vi "UHR-Fleezers Control (host) - 11.9.vi"() -> ()   [LabVIEW 2014] (continued)
                n2362 = call "IMAQ Overlay Oval"("Color"=u32 16711680, "Bounding Rectangle"=w3380, "Image"=w3383) -> ("Image Out"=w3381:T2)  [unwired: 7 in, 1 out]
              }
            }
            "Primary Video Display" <- w3352
          }
        }
        n2363 = node-c288(w3314) -> ()  [unwired: 1 out]
      }
      n2364 = node-c288(w3298) -> ()  [unwired: 1 out]
      n2365 = call "DMR_CloseDevice2.vi"("driver handle IN"=w3303) -> ()  [unwired: 1 in, 4 out]
    }
    frame #4 {
      n2366 = call "DMR_Close.vi"() -> ()  [unwired: 1 out]
    }
  }
  n2367 = local write "Offset (nm)"(0.0 ("Offset (nm)")) -> ()
  n2368 = local write "Bead Mean (nm)"(0.0 ("Bead Mean (nm)")) -> ()
  n2369 = local write "Total Volume\nFlowed P1 (uL)"(w14) -> ()
  n2370 = local write "Total Volume\nFlowed Samp (uL)"(w14) -> ()
  n2371 = local write "Total Volume\nFlowed P3 (uL)"(w14) -> ()
  n2372 = node-c288(i64 1 ("Period"), 1 ("Processor")) -> (w193:T21)  [unwired: 2 out]
  n2373 = timed-loop "Acquire Data" {
    tunnel: w20 -> [w3749]
    tunnel: w69 -> [w3748]
    tunnel: [w3778] -> w286
    tunnel: [w3773] -> w284
    timing: w193 -> [_]
    timing-out: [_] -> w192
    tunnel: w88 -> [w3588]
    stop <- "Stop All" stop-if-true
    w3506 = "Initialize"
    w3575 = "NI_ChannelName" ("name")
    # "I think that the conversion\nfrom 'wiggle amp' to nm\nis 0.277 nm/input. So, 1000\nfor an input is 277 nm."
    n2374 = node-c288() -> ()  [unwired: 2 out]
    n2375 = First Call?() -> (First Call?: T/F=w3541:bool)
    n2376 = Or(x="Reset", y=w3541) -> (x .or. y?=w3542:bool)
    n2377 = local read "Flushing P1"() -> (w3461:bool)
    n2378 = case "Reset data stream" shown="True" w3542 {
      tunnel: w3749 -> [w4816 w4824]
      tunnel: w3748 -> [w4815 w4823]
      tunnel: [w4816 w4818] -> w3454
      tunnel: [w4815 w4817] -> w3744
      frame False {
      }
      frame True {
        w4821 = TRUE ("AI to FIFO")
        n2379 = local write "Overflow (data lost)"(FALSE ("Overflow (data lost)")) -> ()
        n2380 = call "reset FPGA DMA.vi"("error in"=w4823, "FPGA VI Reference In"=w4824) -> ("error out"=w4819:errorcluster, "FPGA VI Reference Out"=w4820:T19)
        n2381 = xnode "Read/Write Control"("FPGA VI Reference In"=w4820, "error in"=w4819, "AI to FIFO"=w4821, "APD to FIFO"=w4821) -> ("FPGA VI Reference Out"=w4818:T19, "error out"=w4817:errorcluster)
      }
    }
    n2382 = case shown="True" w3461 {
      frame False {
      }
      frame True {
        n2383 = local read "Flush rate (uL/m) P1"() -> (w3851:dbl)
        n2384 = local read "HP1 Flush Time (s)"() -> (w3857:dbl)
        n2385 = local read "DMA Update Period (s)"() -> (w3844:dbl)
        n2386 = Divide(x=w3851, y=60.0) -> (x/y=w3843:dbl)
        n2387 = feedback #4(0.0) -> (w3846:dbl)
        n2388 = Divide(x=w3857, y=w3844) -> (x/y=w3849:dbl)
        n2389 = feedback #5(0) -> (w3855:i32)
        n2390 = Increment(x=w3855) -> (x+1=w3848:i32)
        n2391 = Multiply(x=w3844, y=w3843) -> (x*y=w3842:dbl)
        n2392 = Greater?(x=w3848, y=w3849) -> (0:w3854:bool)
        n2393 = Compound Arithmetic op=MULTIPLY(w3844, w3848, w3843) -> (→"P1 Flush Volume (uL)":dbl)
        n2394 = Divide(x=w3848, y=w3849) -> (x/y=→"P1 Flushing Bar":dbl)
        n2395 = Add(x=w3842, y=w3846) -> (x+y=w3845:dbl)
        "Total Volume\nFlowed P1 (uL)" <- w3845
        n2396 = feedback-in #4(w3845) -> ()
        n2397 = case shown="True" w3854 {
          tunnel: w3848 -> [w3858 _]
          tunnel: [w3858 0] -> w3853
          frame False {
          }
          frame True {
            w3859 = FALSE ("Flushing P1")
            n2398 = local write "Inject Pump 1"(w3859) -> ()
            n2399 = local write "Flushing P1"(w3859) -> ()
            n2400 = property on="Clear Volume P1" class="Bool (strict)"("Val(Sgnl)"=TRUE ("Value (Signaling)")) -> ()  [unwired: 2 in, 2 out]
          }
        }
        n2401 = feedback-in #5(w3853) -> ()
      }
    }
    n2402 = Or(x="Start AOD Scan", y="Trap Raster Scan") -> (x .or. y?=w3696:bool)
    n2403 = case "Start AOM raster scan" shown="True" w3696 {
      tunnel: w3454 -> [w4666 w4676]
      tunnel: w3744 -> [w4665 w4675]
      tunnel: [w4666 w4669] -> w3446
      tunnel: [w4665 w4668] -> w3743
      frame False {
      }
      frame True {
        n2404 = case shown="True" "Restart DMA? (AOD)" {
          tunnel: [w4714 w4716] -> w4670
          tunnel: [w4713 w4715] -> w4671
          tunnel: w4676 -> [w4714 w4718]
          tunnel: w4675 -> [w4713 w4717]
          frame False {
          }
          frame True {
            n2405 = local write "Overflow (data lost)"(FALSE ("Overflow (data lost)")) -> ()
            n2406 = call "reset FPGA DMA.vi"("error in"=w4717, "FPGA VI Reference In"=w4718) -> ("error out"=w4715:errorcluster, "FPGA VI Reference Out"=w4716:T19)
          }
        }
        n2407 = local write "Trap Raster Scan"(FALSE ("Trap Raster Scan")) -> ()
        n2408 = case shown="False" "Move MCL Also?" {
          tunnel: w4671 -> [w4680 w4708]
          tunnel: w4670 -> [w4681 w4709]
          tunnel: [w4679 w4712] -> w4669
          tunnel: [w4678 w4711] -> w4668
          frame False {
            w4677 = TRUE ("AI to FIFO")
            n2409 = xnode "Read/Write Control"("FPGA VI Reference In"=w4681, "error in"=w4680, "AI to FIFO"=w4677, "APD to FIFO"=w4677, "Start scan"=w4677) -> ("FPGA VI Reference Out"=w4679:T19, "error out"=w4678:errorcluster)
          }
          frame True {
            w4705 = FALSE ("1D or 2D Scan?")
            w4710 = TRUE ("AI to FIFO")
            # "Count for MCL loop"
            # "N total cycles"
            # "N steps"
            # "V_int"
            n2410 = local read "Scan Range (nm)"() -> (w4687:dbl)
            n2411 = local read "Number of F/B Scans (AOD)"() -> (w4704:u16)
            n2412 = Sign(1:w4687) -> (0:w4686:dbl)
            n2413 = Compound Arithmetic op=MULTIPLY(w4687, "MCL Step Position Ratio", "MCL/AOM Scale Tweak") -> (w4691:dbl)
            n2414 = Negate(x=w4686) -> (-x=w4683:dbl)
            n2415 = Multiply(x=w4683, y="MCL Step Increment (V_int)") -> (x*y=w4685:dbl)
            n2416 = Divide(x=w4691, y="MCL X Cal (nm/V)") -> (x/y=w4697:dbl)
            n2417 = Multiply(x=32767.0 ("y"), y=w4697) -> (x*y=w4703:dbl)
            n2418 = local read "Total Counts (ticks)"() -> (w4688:u32)
            n2419 = local read "Cycles/step (AOD)"() -> (w4699:u64)
            n2420 = local read "Scan steps (AOD)"() -> (w4700:u64)
            n2421 = Divide(x=w4703, y=10.0) -> (x/y=w4696:dbl)
            n2422 = Divide(x=w4696, y="MCL Step Increment (V_int)") -> (x/y=w4694:dbl)
            n2423 = Absolute Value(x=w4694) -> (abs(x)=w4682:dbl)
            n2424 = Compound Arithmetic op=MULTIPLY(w4700, w4699, w4688) -> (w4695:u64)
            n2425 = local write "wait to reset values"(w4710) -> ()
            n2426 = local write "MCL Scanning"(w4710) -> ()
            n2427 = Divide(x=w4695, y=w4682) -> (x/y=w4692:dbl)
            "MCL Count" <- w4692
            n2428 = xnode "Read/Write Control"("FPGA VI Reference In"=w4709, "error in"=w4708, "Scan steps (MCL)"=w4682, "Number of scans (MCL)"=w4704, "Cycles per step (MCL)"=u64 1, "Scan freq.  increment (MCL)"=w4685, "1D or 2D Scan?"=w4705, "MCL Scan Axis"=w4705, "Cont. Scan (MCL)"=w4705, "MCL count"=w4692) -> ("FPGA VI Reference Out"=w4707:T19, "error out"=w4706:errorcluster)
            n2429 = xnode "Read/Write Control"("FPGA VI Reference In"=w4707, "error in"=w4706, "AI to FIFO"=w4710, "APD to FIFO"=w4710, "Start scan"=w4710, "Start scan (MCL)"=w4710) -> ("FPGA VI Reference Out"=w4712:T19, "error out"=w4711:errorcluster)
          }
        }
        "Raster Scanning..." <- TRUE ("Scanning...")
      }
    }
    n2430 = local read "Flushing P3"() -> (w3462:bool)
    n2431 = case "Keep track of when Harvard Pump 3 is done flushing" shown="True" w3462 {
      frame False {
      }
      frame True {
        n2432 = local read "Flush rate (uL/m) P3"() -> (w3870:dbl)
        n2433 = local read "DMA Update Period (s)"() -> (w3864:dbl)
        n2434 = local read "HP3 Flush Time (s)"() -> (w3878:dbl)
        n2435 = Divide(x=w3870, y=60.0) -> (x/y=w3865:dbl)
        n2436 = feedback #6(0) -> (w3876:i32)
        n2437 = Increment(x=w3876) -> (x+1=w3871:i32)
        n2438 = Divide(x=w3878, y=w3864) -> (x/y=w3872:dbl)
        n2439 = Multiply(x=w3864, y=w3865) -> (x*y=w3863:dbl)
        n2440 = Greater?(x=w3871, y=w3872) -> (0:w3875:bool)
        n2441 = feedback #7(0.0) -> (w3866:dbl)
        n2442 = Compound Arithmetic op=MULTIPLY(w3864, w3871, w3865) -> (→"P3 Flush Volume (uL)":dbl)
        n2443 = case shown="True" w3875 {
          tunnel: w3871 -> [w3879 _]
          tunnel: [w3879 0] -> w3874
          frame False {
          }
          frame True {
            w3880 = FALSE ("Flushing P3")
            n2444 = local write "Inject Pump 3"(w3880) -> ()
            n2445 = local write "Flushing P3"(w3880) -> ()
            n2446 = property on="Clear Volume P3" class="Bool (strict)"("Val(Sgnl)"=TRUE ("Value (Signaling)")) -> ()  [unwired: 2 in, 2 out]
          }
        }
        n2447 = feedback-in #6(w3874) -> ()
        n2448 = Divide(x=w3871, y=w3872) -> (x/y=→"P3 Flushing Bar":dbl)
        n2449 = Add(x=w3863, y=w3866) -> (x+y=w3867:dbl)
        "Total Volume\nFlowed P3 (uL)" <- w3867
        n2450 = feedback-in #7(w3867) -> ()
      }
    }
    n2451 = And(x="Save scans", y=w3696) -> (x .and. y?=w3742:bool)
    n2452 = local read "Flushing samp"() -> (w3455:bool)
    n2453 = case shown="True" w3455 {
      frame False {
      }
      frame True {
        n2454 = local read "DMA Update Period (s)"() -> (w3823:dbl)
        n2455 = local read "Flush rate (mL/m)"() -> (w3835:dbl)
        n2456 = local read "Samp Flush Time (s)"() -> (w3836:dbl)
        n2457 = Divide(x=w3835, y=60.0) -> (x/y=w3822:dbl)
        n2458 = feedback #8(0) -> (w3828:i32)
        n2459 = Increment(x=w3828) -> (x+1=w3827:i32)
        n2460 = Divide(x=w3836, y=w3823) -> (x/y=w3832:dbl)
        n2461 = Multiply(x=w3823, y=w3822) -> (x*y=w3821:dbl)
        n2462 = Greater?(x=w3827, y=w3832) -> (0:w3831:bool)
        n2463 = feedback #9(0.0) -> (w3824:dbl)
        n2464 = Compound Arithmetic op=MULTIPLY(w3823, w3827, w3822) -> (→"Samp Volume (uL)":dbl)
        n2465 = Divide(x=w3827, y=w3832) -> (x/y=→"Samp flush bar":dbl)
        n2466 = case shown="True" w3831 {
          tunnel: [w3837 0] -> w3830
          tunnel: w3827 -> [w3837 _]
          frame False {
          }
          frame True {
            w3840 = FALSE ("Flushing samp")
            n2467 = local write "Sample Channel\nFlow"(w3840) -> ()
            n2468 = local write "Flushing samp"(w3840) -> ()
            n2469 = property on="Clear Volume" class="Bool (strict)"("Val(Sgnl)"=TRUE) -> ()  [unwired: 2 in, 2 out]
          }
        }
        n2470 = feedback-in #8(w3830) -> ()
        n2471 = Add(x=w3821, y=w3824) -> (x+y=w3825:dbl)
        "Total Volume\nFlowed Samp (uL)" <- w3825
        n2472 = feedback-in #9(w3825) -> ()
      }
    }
    n2473 = Compound Arithmetic op=OR("Start MCL Scan", "Confocal\nImage", "Confocal\nLinescan") -> (w3694:bool)
    n2474 = And(x="Save Data (MCL)", y=w3694) -> (x .and. y?=w3741:bool)
    n2475 = case "Start MCL raster scan" shown="True" w3694 {
      tunnel: w3446 -> [w4283 w4299]
      tunnel: w3743 -> [w4282 w4298]
      tunnel: [w4283 w4294] -> w3453
      tunnel: [w4282 w4293] -> w3451
      tunnel: [FALSE w4292] -> w3727
      tunnel: "Start MCL Scan" -> [_ w4287]
      tunnel: "Confocal\nImage" -> [_ w4286]
      tunnel: "Confocal\nLinescan" -> [_ _]
      frame False {
      }
      frame True {
        w4292 = TRUE
        n2476 = case shown="True" "Restart DMA? (MCL)" {
          tunnel: [w4344 w4346] -> w4297
          tunnel: [w4343 w4345] -> w4296
          tunnel: w4299 -> [w4344 w4349]
          tunnel: w4298 -> [w4343 w4348]
          frame False {
          }
          frame True {
            n2477 = call "reset FPGA DMA.vi"("error in"=w4348, "FPGA VI Reference In"=w4349) -> ("error out"=w4345:errorcluster, "FPGA VI Reference Out"=w4346:T19)
            n2478 = local write "Overflow (data lost)"(FALSE ("Overflow (data lost)")) -> ()
          }
        }
        n2479 = case shown="False" w4287 {
          selector: w4287 -> [_ w4303]
          tunnel: w4286 -> [w4302 _]
          tunnel: [w4302 w4303] -> w4285
          frame False {
            n2480 = property on="2D or 1D Scan" class="Bool (strict)"("Val(Sgnl)"=w4302) -> ()  [unwired: 2 in, 2 out]
            n2481 = property on="Confocal\nImage" class="Bool (strict)"("Value"=FALSE ("Start Confocal Map")) -> ()  [unwired: 2 in, 2 out]
          }
          frame True {
          }
        }
        n2482 = local write "MCL Scanning"(w4292) -> ()
        n2483 = local read "AO1"() -> (w4289:dbl)
        n2484 = local read "AO2"() -> (w4288:dbl)
        n2485 = case shown="True" "Center Scan" {
          tunnel: w4297 -> [w4310 w4342]
          tunnel: w4296 -> [w4309 w4341]
          tunnel: [w4308 w4340] -> w4294
          tunnel: [w4307 w4339] -> w4293
          tunnel: [w4305 w4326] -> w4291
          tunnel: [w4304 w4325] -> w4290
          tunnel: w4289 -> [w4305 w4331]
          tunnel: w4288 -> [w4304 w4334]
          tunnel: w4285 -> [_ _]
          frame False {
            w4306 = TRUE ("AI to FIFO")
            n2486 = xnode "Read/Write Control"("FPGA VI Reference In"=w4310, "error in"=w4309, "AI to FIFO"=w4306, "APD to FIFO"=w4306, "Start scan (MCL)"=w4306) -> ("FPGA VI Reference Out"=w4308:T19, "error out"=w4307:errorcluster)
          }
          frame True {
            w4338 = TRUE ("AI to FIFO")
            n2487 = local read "Scan steps (MCL)"() -> (w4317:u64)
            n2488 = local read "Scan lines (y)"() -> (w4313:u64)
            n2489 = local read "Fast Scan Dir"() -> (w4324:bool)
            n2490 = local read "Actual MCL Inc (V)"() -> (w4314:dbl)
            n2491 = Decrement(x=w4313) -> (x-1=w4312:u64)
            n2492 = Decrement(x=w4317) -> (x-1=w4316:u64)
            n2493 = Multiply(x=w4314, y=w4312) -> (x*y=w4311:dbl)
            n2494 = Divide(x=w4311, y=2.0) -> (x/y=w4321:dbl)
            n2495 = Multiply(x=w4314, y=w4316) -> (x*y=w4315:dbl)
            n2496 = Divide(x=w4315, y=2.0) -> (x/y=w4320:dbl)
            n2497 = Select(t=w4320, s=w4324, f=w4321) -> (s? t:f=w4319:dbl)
            n2498 = Select(t=w4321, s=w4324, f=w4320) -> (s? t:f=w4323:dbl)
            n2499 = Subtract(x=w4331, y=w4323) -> (x-y=w4322:dbl)
            n2500 = Subtract(x=w4334, y=w4319) -> (x-y=w4318:dbl)
            n2501 = local read "2D or 1D Scan"() -> (w4336:bool)
            n2502 = Not(x=w4324) -> (.not. x?=w4330:bool)
            n2503 = Not(x=w4336) -> (.not. x?=w4332:bool)
            n2504 = And(x=w4324, y=w4332) -> (x .and. y?=w4333:bool)
            n2505 = And(x=w4332, y=w4330) -> (x .and. y?=w4335:bool)
            n2506 = Select(t=w4334, s=w4335, f=w4318) -> (s? t:f=w4325:dbl)
            n2507 = Select(t=w4331, s=w4333, f=w4322) -> (s? t:f=w4326:dbl)
            n2508 = call "Volt to I16.vi"("Voltage In"=w4326) -> ("I16 Voltage Out"=w4329:i16)
            n2509 = call "Volt to I16.vi"("Voltage In"=w4325) -> ("I16 Voltage Out"=w4328:i16)
            n2510 = xnode "Read/Write Control"("FPGA VI Reference In"=w4342, "error in"=w4341, "AI to FIFO"=w4338, "APD to FIFO"=w4338, "Start scan (MCL)"=w4338, "AO1"=w4329, "AO2"=w4328) -> ("FPGA VI Reference Out"=w4340:T19, "error out"=w4339:errorcluster)
          }
        }
        "Initial Y" <- w4291
        "Initial X" <- w4290
        n2511 = local write "Tab Control 6"(T3."Imaging" ("Tab Control 6")) -> ()
        "wait to reset values" <- w4292
      }
    }
    n2512 = xnode "Read/Write Control"("FPGA VI Reference In"=w3446) -> ("Green Enabled"=w3445)  [unwired: 1 in, 2 out]
    n2513 = local write "Grn enabl"(w3445) -> ()
    n2514 = case shown="True" "Wiggle" {
      selector: "Wiggle" -> [w3794 _]
      tunnel: w3453 -> [w3796 w3809]
      tunnel: [w3793 w3812] -> w3452
      tunnel: w3451 -> [w3795 w3807]
      tunnel: [w3792 w3811] -> w3450
      frame False {
        n2515 = xnode "Read/Write Control"("FPGA VI Reference In"=w3796, "error in"=w3795, "Wiggle trap 1"=w3794) -> ("FPGA VI Reference Out"=w3793:T19, "error out"=w3792:errorcluster)
      }
      frame True {
        w3801 = FALSE ("Abort wiggle")
        w3805 = TRUE
        n2516 = local read "Restart DMA? (AOD)"() -> (w3810:bool)
        n2517 = case shown="True" w3810 {
          tunnel: w3809 -> [w3814 w3819]
          tunnel: [w3814 w3818] -> w3808
          tunnel: w3807 -> [w3813 w3817]
          tunnel: [w3813 w3816] -> w3806
          frame False {
          }
          frame True {
            n2518 = local write "Overflow (data lost)"(FALSE) -> ()
            n2519 = call "reset FPGA DMA.vi"("error in"=w3817, "FPGA VI Reference In"=w3819) -> ("error out"=w3816:errorcluster, "FPGA VI Reference Out"=w3818:T19)
          }
        }
        n2520 = local write "Wiggle"(FALSE) -> ()
        n2521 = xnode "Read/Write Control"("FPGA VI Reference In"=w3808, "error in"=w3806, "AI to FIFO"=w3805, "APD to FIFO"=w3805, "Wiggle trap 1"="Wiggle T1", "Wiggle freq 1 (Hz)"="Wiggle freq 1 (Hz)", "Wiggle amp 1"="Wiggle amp 1 (units?)", "Abort wiggle 1"=w3801, "Wiggle trap 2"="Wiggle T2", "Abort wiggle 2"=w3801, "Wiggle freq 2 (Hz)"="Wig Freq 2 (Hz)", "Wiggle amp 2"="Wig amp 2") -> ("FPGA VI Reference Out"=w3812:T19, "error out"=w3811:errorcluster)
      }
    }
    n2522 = local read "Trap Pos Elements/DMA read"() -> (w3584:u32)
    n2523 = local read "Trap AI Elements/DMA read"() -> (w3657:u32)
    n2524 = local read "APD Elements/DMA read"() -> (w3623:u32)
    n2525 = xnode "Get APD Data"("FPGA VI Reference In"=w3452, "error in"=w3450, "Number of Elements"=w3623, "Timeout (ms)"=-1) -> ("Data"=w3622:u32[], "Elements Remaining"=→"APD FIFO Elements Remaining":u32)  [unwired: 2 out]
    n2526 = xnode "Invoke Method"("FPGA VI Reference In"=w3452, "error in"=w3450, "Number of Elements"=w3584, "Timeout (ms)"=-1) -> ("Data"=w3548:u16[], "Elements Remaining"=→"Trap Pos FIFO El Remaining":u32)  [unwired: 2 out]
    n2527 = xnode "Get Trap Data"("FPGA VI Reference In"=w3452, "error in"=w3450, "Number of Elements"=w3657, "Timeout (ms)"=-1 ("Timeout")) -> ("FPGA VI Reference Out"=w3483:T19, "error out"=w3482:errorcluster, "Data"=w3549:i16[], "Elements Remaining"=w3786:u32)
    "FIFO El. Rem." <- w3786
    n2528 = local read "Trap AI FIFO Depth"() -> (w3788:u32)
    n2529 = Subtract(x=w3788, y=w3657) -> (x-y=w3787:u32)
    n2530 = Decimate 1D Array(w3548) -> (w3545:u16[], w3547:u16[], w3546:u16[])
    n2531 = Divide(x=w3786, y=w3787) -> (x/y=w3785:dbl)
    "Buffer Status" <- w3785
    n2532 = To Unsigned Long Integer(number=w3545) -> (unsigned 32bit integer=w3544:u32[])
    n2533 = Join Numbers(hi=w3547, lo=w3546) -> ((hi.lo)=w3543:u32[])
    n2534 = Equal?(x=w3785, y=1.0) -> (x = y?=w3783:bool)
    n2535 = Join Numbers(hi=w3544, lo=w3543) -> ((hi.lo)=w3537:u64[])
    n2536 = call "IR AOM word to freq - vec.vi"("Frequency Word In (double vec)"=w3537) -> ("Frequency Out"=w3583:dbl[])
    n2537 = case "Alert buffer overflow" shown="True" w3783 {
      frame False {
      }
      frame True {
        n2538 = call <vilib>:"Beep.vi"() -> ()  [unwired: 3 in, 9 out]
        "Overflow (data lost)" <- TRUE ("Overflow (data lost)")
      }
    }
    n2539 = Decimate 1D Array(w3583) -> (w3582:dbl[], w3581:dbl[])
    n2540 = Build Array(w3582, w3581) -> (w3580:dbl[][])
    n2541 = local read "Trap Sets"() -> (w3656:u32)
    n2542 = case "Deinterlace trap data, average down PSD" shown="2" w3656 {
      tunnel: w3549 -> [w4379 w4444]
      tunnel: [w4376 w4441] -> w3649
      tunnel: [w4379 w4443] -> w3540
      tunnel: "Detector Type" -> [w4378 w4439]
      tunnel: [w4377 w4442] -> w3648
      tunnel: [w4375 w4440] -> w3760
      frame 1, Default {
        n2543 = Divide(x=w4379, y=3276.7) -> (x/y=w4380:dbl[])
        n2544 = Decimate 1D Array(w4380) -> (w4389:dbl[], w4388:dbl[], w4387:dbl[], w4386:dbl[], w4385:dbl[], w4384:dbl[], w4383:dbl[], w4382:dbl[])
        n2545 = case shown="\"IR-QPD + PSD + FB-QPD position\"" w4378 {
          tunnel: w4389 -> [w4413 w4438]
          tunnel: w4388 -> [w4412 w4437]
          tunnel: w4387 -> [w4397 w4415]
          tunnel: w4386 -> [w4398 w4425]
          tunnel: w4385 -> [w4411 w4436]
          tunnel: w4384 -> [w4410 w4435]
          tunnel: w4383 -> [w4394 w4416]
          tunnel: w4382 -> [w4393 w4414]
          tunnel: [w4392 w4422] -> w4377
          tunnel: [w4391 w4421] -> w4376
          tunnel: [w4390 w4420] -> w4375
          frame "IR-QPD + PSD + FB-QPD", Default {
            w4390 = 0  # Channel pattern
            n2546 = Divide(x=w4413, y=w4398) -> (x/y=w4400:dbl[])
            n2547 = Divide(x=w4412, y=w4398) -> (x/y=w4399:dbl[])
            n2548 = Divide(x=w4411, y=w4394) -> (x/y=w4396:dbl[])
            n2549 = Divide(x=w4410, y=w4393) -> (x/y=w4395:dbl[])
            n2550 = Build Array(w4400, w4399, w4398, w4397, w4396, w4395, w4394, w4393) -> (w4391:dbl[][])
            n2551 = Bundle("T1 Y", "T1 X", "T1 Sum", "FB Sum", "PSD Y", "PSD X", "PSD Y Sum", "PSD X Sum") -> (w4409:T41)  [unwired: 1 out]
            n2552 = Cluster To Array(cluster=w4409) -> (array=w4392:string[])
          }
          frame "IR-QPD + PSD + FB-QPD position" {
            w4420 = 3  # Channel pattern
            n2553 = Negate(x=w4416) -> (-x=w4417:dbl[])
            n2554 = Divide(x=w4438, y=w4425) -> (x/y=w4427:dbl[])
            n2555 = Divide(x=w4437, y=w4425) -> (x/y=w4426:dbl[])
            n2556 = Divide(x=w4436, y=w4416) -> (x/y=w4424:dbl[])
            n2557 = Divide(x=w4435, y=w4417) -> (x/y=w4423:dbl[])
            n2558 = Build Array(w4427, w4426, w4425, w4414, w4415, w4424, w4423, w4416) -> (w4421:dbl[][])
            n2559 = Bundle("T1 Y", "T1 X", "T1 Sum", "FB X", "FB Sum", "PSD Y", "PSD X", "PSD Y Sum") -> (w4434:T41)  [unwired: 1 out]
            n2560 = Cluster To Array(cluster=w4434) -> (array=w4422:string[])
          }
        }
      }
      frame 2 {
        n2561 = case shown="\"IR-QPD + PSD + FB-QPD\", Default" w4439 {
          tunnel: w4444 -> [w4506 w4573 w4644]
          tunnel: [w4445 w4564 w4575] -> w4443
          tunnel: [w4472 w4555 w4622] -> w4442
          tunnel: [w4471 w4518 w4589] -> w4441
          tunnel: [w4465 w4553 w4620] -> w4440
          frame "IR-QPD + PSD + FB-QPD", Default {
            w4465 = 1  # Channel pattern
            # "time average x2 the 4th signal and the 4 psd signals (detection laser)"
            # "deinterlace 3 signals from qpd"
            n2562 = Decimate 1D Array(w4506) -> (w4505:i16[], w4504:i16[], w4470:i16[], w4503:i16[], w4493:i16[], w4491:i16[], w4490:i16[], w4488:i16[])
            n2563 = Decimate 1D Array(w4470) -> (w4469:i16[], w4468:i16[])
            n2564 = Decimate 1D Array(w4505) -> (w4502:i16[], w4474:i16[])
            n2565 = Decimate 1D Array(w4504) -> (w4501:i16[], w4499:i16[])
            n2566 = Decimate 1D Array(w4503) -> (w4500:i16[], w4498:i16[])
            n2567 = call "downsample 1D array - double.vi"("Ave N"=2.0, "Array In"=w4493) -> ("Array Out"=w4492:dbl[])  [unwired: 1 out]
            n2568 = call "downsample 1D array - double.vi"("Ave N"=2.0, "Array In"=w4491) -> ("Array Out"=w4473:dbl[])  [unwired: 1 out]
            n2569 = call "downsample 1D array - double.vi"("Ave N"=2.0, "Array In"=w4490) -> ("Array Out"=w4489:dbl[])  [unwired: 1 out]
            n2570 = call "downsample 1D array - double.vi"("Ave N"=2.0, "Array In"=w4488) -> ("Array Out"=w4487:dbl[])  [unwired: 1 out]
            n2571 = Interleave 1D Arrays(w4502, w4501, w4500, w4474, w4499, w4498, w4469, w4468, w4492, w4473, w4489, w4487) -> (w4486:dbl[])
            n2572 = Divide(x=w4486, y=3276.7) -> (x/y=w4485:dbl[])
            n2573 = Decimate 1D Array(w4485) -> (w4484:dbl[], w4483:dbl[], w4482:dbl[], w4481:dbl[], w4480:dbl[], w4479:dbl[], w4467:dbl[], w4466:dbl[], w4478:dbl[], w4477:dbl[], w4476:dbl[], w4475:dbl[])
            n2574 = Divide(x=w4484, y=w4482) -> (x/y=w4452:dbl[])
            n2575 = Divide(x=w4483, y=w4482) -> (x/y=w4451:dbl[])
            n2576 = Divide(x=w4481, y=w4479) -> (x/y=w4450:dbl[])
            n2577 = Divide(x=w4480, y=w4479) -> (x/y=w4449:dbl[])
            n2578 = Divide(x=w4478, y=w4476) -> (x/y=w4448:dbl[])
            n2579 = Divide(x=w4477, y=w4475) -> (x/y=w4447:dbl[])
            n2580 = Build Array(w4452, w4451, w4482, w4450, w4449, w4479, w4467, w4466, w4448, w4447, w4476, w4475) -> (w4471:dbl[][])
            n2581 = Bundle("T1 Y", "T1 X", "T1 Sum", "T2 Y", "T2 X", "T2 Sum", "T1 FB Sum", "T2 FB Sum", "PSD Y", "PSD X", "PSD Y Sum", "PSD X Sum") -> (w4453:T42)  [unwired: 1 out]
            n2582 = To Word Integer(number=w4486) -> (16bit integer=w4445:i16[])
            n2583 = Cluster To Array(cluster=w4453) -> (array=w4472:string[])
          }
          frame "IR-QPD + PSD + FB-QPD X position" {
            w4553 = 2  # Channel pattern
            # "time average x2 the 3 psd signals (detection laser)"
            # "deinterlace 3 signals from qpds"
            n2584 = Decimate 1D Array(w4573) -> (w4572:i16[], w4571:i16[], w4554:i16[], w4570:i16[], w4516:i16[], w4513:i16[], w4510:i16[], w4541:i16[])
            n2585 = Decimate 1D Array(w4554) -> (w4539:i16[], w4537:i16[])
            n2586 = Decimate 1D Array(w4572) -> (w4569:i16[], w4556:i16[])
            n2587 = Decimate 1D Array(w4571) -> (w4568:i16[], w4566:i16[])
            n2588 = Decimate 1D Array(w4570) -> (w4567:i16[], w4565:i16[])
            n2589 = Decimate 1D Array(w4541) -> (w4540:i16[], w4538:i16[])
            n2590 = call "downsample 1D array - I16.vi"("Ave N"=2.0, "Array In"=w4516) -> ("Array Out"=w4514:i16[])  [unwired: 1 in]
            n2591 = call "downsample 1D array - I16.vi"("Ave N"=2.0, "Array In"=w4510) -> ("Array Out"=w4508:i16[])  [unwired: 1 in]
            n2592 = call "downsample 1D array - I16.vi"("Ave N"=2.0, "Array In"=w4513) -> ("Array Out"=w4511:i16[])  [unwired: 1 in]
            n2593 = Interleave 1D Arrays(w4569, w4568, w4567, w4556, w4566, w4565, w4540, w4539, w4538, w4537, w4514, w4511, w4508) -> (w4564:i16[])
            n2594 = Divide(x=w4564, y=3276.7) -> (x/y=w4563:dbl[])
            n2595 = Decimate 1D Array(w4563) -> (w4562:dbl[], w4561:dbl[], w4560:dbl[], w4559:dbl[], w4558:dbl[], w4557:dbl[], w4529:dbl[], w4527:dbl[], w4526:dbl[], w4524:dbl[], w4523:dbl[], w4522:dbl[], w4519:dbl[])
            n2596 = Negate(x=w4519) -> (-x=w4517:dbl[])
            n2597 = Divide(x=w4523, y=w4519) -> (x/y=w4521:dbl[])
            n2598 = Divide(x=w4522, y=w4517) -> (x/y=w4520:dbl[])
            n2599 = Divide(x=w4562, y=w4560) -> (x/y=w4545:dbl[])
            n2600 = Divide(x=w4561, y=w4560) -> (x/y=w4544:dbl[])
            n2601 = Divide(x=w4559, y=w4557) -> (x/y=w4543:dbl[])
            n2602 = Divide(x=w4558, y=w4557) -> (x/y=w4542:dbl[])
            n2603 = Divide(x=w4529, y=w4527) -> (x/y=w4528:dbl[])
            n2604 = Divide(x=w4526, y=w4524) -> (x/y=w4525:dbl[])
            n2605 = Build Array(w4545, w4544, w4560, w4543, w4542, w4557, w4528, w4527, w4525, w4524, w4521, w4520, w4519) -> (w4518:dbl[][])
            n2606 = Bundle("T1 Y", "T1 X", "T1 Sum", "T2 Y", "T2 X", "T2 Sum", "T1 FB X", "T1 FB Sum", "T2 FB X", "T2 FB Sum", "PSD Y", "PSD X", "PSD Y Sum") -> (w4546:T43)  [unwired: 1 out]
            n2607 = Cluster To Array(cluster=w4546) -> (array=w4555:string[])
          }
          frame "IR-QPD + PSD + FB-QPD XY positions" {
            w4620 = 4  # Channel pattern
            # "time average x2 the 3 psd signals (detection laser)"
            # "deinterlace 3 signals from qpds"
            n2608 = Decimate 1D Array(w4644) -> (w4643:i16[], w4642:i16[], w4621:i16[], w4641:i16[], w4587:i16[], w4633:i16[], w4632:i16[], w4609:i16[])
            n2609 = Decimate 1D Array "Feedback Sum"(w4621) -> (w4605:i16[], w4603:i16[])
            n2610 = Decimate 1D Array "QPD Y"(w4643) -> (w4640:i16[], w4623:i16[])
            n2611 = Decimate 1D Array "QPD X"(w4642) -> (w4639:i16[], w4637:i16[])
            n2612 = Decimate 1D Array "Feedback Y"(w4587) -> (w4586:i16[], w4585:i16[])
            n2613 = Decimate 1D Array "QPD Sum"(w4641) -> (w4638:i16[], w4636:i16[])
            n2614 = Decimate 1D Array "Feedback X"(w4609) -> (w4606:i16[], w4604:i16[])
            n2615 = call "downsample 1D array - double.vi"("Ave N"=2.0, "Array In"=w4633) -> ("Array Out"=w4608:dbl[])  [unwired: 1 out]
            n2616 = call "downsample 1D array - double.vi"("Ave N"=2.0, "Array In"=w4632) -> ("Array Out"=w4607:dbl[])  [unwired: 1 out]
            n2617 = Interleave 1D Arrays(w4640, w4639, w4638, w4623, w4637, w4636, w4586, w4606, w4605, w4585, w4604, w4603, w4608, w4607) -> (w4631:dbl[])
            n2618 = Divide(x=w4631, y=3276.7) -> (x/y=w4630:dbl[])
            n2619 = Decimate 1D Array(w4630) -> (w4629:dbl[], w4628:dbl[], w4627:dbl[], w4626:dbl[], w4625:dbl[], w4624:dbl[], w4582:dbl[], w4596:dbl[], w4580:dbl[], w4581:dbl[], w4594:dbl[], w4578:dbl[], w4592:dbl[], w4590:dbl[])
            n2620 = Negate(x=w4590) -> (-x=w4588:dbl[])
            n2621 = Divide(x=w4592, y=w4588) -> (x/y=w4591:dbl[])
            n2622 = Divide(x=w4581, y=w4578) -> (x/y=w4577:dbl[])
            n2623 = Divide(x=w4582, y=w4580) -> (x/y=w4579:dbl[])
            n2624 = Divide(x=w4629, y=w4627) -> (x/y=w4613:dbl[])
            n2625 = Divide(x=w4628, y=w4627) -> (x/y=w4612:dbl[])
            n2626 = Divide(x=w4626, y=w4624) -> (x/y=w4611:dbl[])
            n2627 = Divide(x=w4625, y=w4624) -> (x/y=w4610:dbl[])
            n2628 = Divide(x=w4596, y=w4580) -> (x/y=w4595:dbl[])
            n2629 = Divide(x=w4594, y=w4578) -> (x/y=w4593:dbl[])
            n2630 = Build Array(w4613, w4612, w4627, w4611, w4610, w4624, w4579, w4595, w4580, w4577, w4593, w4578, w4591, w4590) -> (w4589:dbl[][])
            n2631 = Bundle("T1 Y", "T1 X", "T1 Sum", "T2 Y", "T2 X", "T2 Sum", "T1 FB Y", "T1 FB X", "T1 FB Sum", "T2 FB Y", "T2 FB X", "T2 FB Sum", "PSD X", "PSD Y Sum") -> (w4576:T44)  [unwired: 1 out]
            n2632 = To Word Integer(number=w4631) -> (16bit integer=w4575:i16[])
            n2633 = Cluster To Array(cluster=w4576) -> (array=w4622:string[])
          }
        }
      }
    }
    "AI labels" <- w3648
    n2634 = Decimate 1D Array(w3622) -> (w3646:u32[], w3590:u32[])
    n2635 = local read "DMA Update Period (s)"() -> (w3658:dbl)
    n2636 = Build Array(w3646, w3590) -> (w3724:u32[][])
    n2637 = local read "Data Period (s)"() -> (w3499:dbl)
    n2638 = local read "BD 1 Frequency 2 (MHz)"() -> (w3532:dbl)
    n2639 = local read "BD 1 Frequency 1 (MHz)"() -> (w3533:dbl)
    n2640 = Decimate 1D Array(w3540) -> (w3563:i16[], w3562:i16[], w3560:i16[], w3559:i16[])  [unwired: 9 out]
    n2641 = To Double Precision Float(number=w3724) -> (double precision float=w3725:dbl[][])
    n2642 = local read "APD Integration Time (s)"() -> (w3603:dbl)
    n2643 = Multiply(x=w3499, y="Trap Pos. Disp. Downsample") -> (x*y=w3497:dbl)
    n2644 = Divide(x=w3563, y=w3562) -> (x/y=w3564:dbl[])
    n2645 = Divide(x=w3560, y=w3559) -> (x/y=w3561:dbl[])
    n2646 = feedback #10(0.0) -> (w3577:dbl)
    n2647 = Add(x=w3658, y=w3577) -> (x+y=w3762:dbl)
    n2648 = feedback-in #10(w3762) -> ()
    n2649 = local read "AOM X Cal (nm/MHz)"() -> (w3530:dbl)
    n2650 = To Time Stamp(1:w3577) -> (0:w3576:timestamp)
    n2651 = Split 1D Array(array=w3564, index="N El. to Ave.") -> (second subarray=w3567:dbl[])  [unwired: 1 out]
    n2652 = Split 1D Array(array=w3561, index="N El. to Ave.") -> (second subarray=w3566:dbl[])  [unwired: 1 out]
    n2653 = Multiply(x=w3499, y="Trap Disp. Downsample") -> (x*y=w3578:dbl)
    "Display Period (s)" <- w3578
    n2654 = for "Trap AI" {
      tunnel: [w4374] -> w3756 mode=indexing
      tunnel: w3576 -> [w4364]
      tunnel: "Trap Disp. Downsample" -> [w4372]
      tunnel: w3649 -> [w4370] mode=indexing
      tunnel: w3499 -> [w4369]
      tunnel: w3648 -> [w4368] mode=indexing
      tunnel: w3575 -> [w4367]
      tunnel: [w4366] -> w3614 mode=indexing
      tunnel: w3578 -> [w4365]
      workers-P: _ -> [_]
      n2655 = Bundle By Name("Y"=w4370, "dt"=w4369) -> (w4371:waveform(dbl))  [unwired: 1 out]
      n2656 = Set Waveform Attribute(5:w4368, 6:w4367, 7:w4371) -> (3:w4366:waveform(dbl))  [unwired: 1 in, 2 out]
      n2657 = call "downsample 1D array - double.vi"("Ave N"=w4372, "Array In"=w4370) -> ("Array Out"=w4373:dbl[])  [unwired: 1 out]
      n2658 = Bundle By Name(cluster=w4366, "t0"=w4364, "Y"=w4373, "dt"=w4365) -> (w4374:waveform(dbl))
    }
    n2659 = Bundle("BD 1 Frequency 1 (MHz)"=w3533, "BD 1 Frequency 2 (MHz)"=w3532) -> (w3534:T45)  [unwired: 1 out]
    n2660 = call-poly <vilib>:"Mean.vi"("X"=w3566) -> ("mean"=w3554:dbl)  [unwired: 1 out]
    n2661 = call-poly <vilib>:"Mean.vi"("X"=w3567) -> ("mean"=w3555:dbl)  [unwired: 1 out]
    n2662 = Reciprocal(x=w3578) -> (1/x=→"Trap Disp. Freq. (Hz)":dbl)
    n2663 = Cluster To Array(cluster=w3534) -> (array=w3531:dbl[])
    n2664 = local read "Trap X AI1 (DMA)"() -> (w3565:T13)
    n2665 = local read "Data points/scans (MCL)"() -> (w3736:dbl)
    n2666 = To Fixed-Point(number=w3554) -> (fixed-point=w3552:fxp<+/-,16,1>)  [unwired: 1 in]
    n2667 = To Fixed-Point(number=w3555) -> (fixed-point=w3553:fxp<+/-,16,1>)  [unwired: 1 in]
    n2668 = Bundle("Trap 1 Pos.", "Trap 2 Pos.") -> (w3574:cluster{string, string})  [unwired: 1 out]
    n2669 = Bundle By Name(cluster=w3565, "Set 1"=w3553, "Set 2"=w3552) -> (→"Trap X AI1 (DMA)":T13)
    n2670 = Cluster To Array(cluster=w3574) -> (array=w3571:string[])
    n2671 = Bundle("APD 1", "APD 2") -> (w3755:cluster{string, string})  [unwired: 1 out]
    n2672 = Select(t=-1.0, s="Negate Y Axis", f=1.0) -> (s? t:f=w3516:dbl)
    n2673 = for "Trap Position" {
      tunnel: w3580 -> [w4008] mode=indexing
      tunnel: "Trap Pos. Disp. Downsample" -> [w4007]
      tunnel: w3497 -> [w4005]
      tunnel: w3576 -> [w4004]
      tunnel: w3575 -> [w4002]
      tunnel: w3571 -> [w4001] mode=indexing
      tunnel: [w4000] -> w3486 mode=indexing
      tunnel: w3531 -> [w3998] mode=indexing
      tunnel: w3530 -> [w3996]
      tunnel: w3516 -> [w3995]
      n2674 = call "downsample 1D array - double.vi"("Ave N"=w4007, "Array In"=w4008) -> ("Array Out"=w4006:dbl[])  [unwired: 1 out]
      n2675 = Subtract(x=w4006, y=w3998) -> (x-y=w3999:dbl[])
      n2676 = Multiply(x=w3996, y=w3999) -> (x*y=w3997:dbl[])
      n2677 = Multiply(x=w3995, y=w3997) -> (x*y=w3994:dbl[])
      n2678 = Bundle By Name("Y"=w3994, "dt"=w4005, "t0"=w4004) -> (w4003:waveform(dbl))  [unwired: 1 out]
      n2679 = Set Waveform Attribute(5:w4001, 6:w4002, 7:w4003) -> (3:w4000:waveform(dbl))  [unwired: 1 in, 2 out]
    }
    n2680 = Cluster To Array(cluster=w3755) -> (array=w3752:string[])
    n2681 = for "APD" {
      tunnel: w3725 -> [w4353] mode=indexing
      tunnel: w3603 -> [w4361]
      tunnel: [w4357] -> w3610 mode=indexing
      tunnel: "APD Disp. Scale" -> [w4358]
      tunnel: w3575 -> [w4356]
      tunnel: w3752 -> [w4355] mode=indexing
      tunnel: "APD Disp. Downsample" -> [w4351]
      tunnel: [w4354] -> w3751
      workers-P: _ -> [_]
      tunnel: w3576 -> [w4350]
      n2682 = call "integrate 1D array interval - double.vi"("Ave N"=w4351, "Array In"=w4353) -> ("Array Out"=w4352:dbl[])  [unwired: 1 out]
      n2683 = Multiply(x=w4361, y=w4351) -> (x*y=w4354:dbl)
      n2684 = Divide(x=w4352, y=w4358) -> (x/y=w4359:dbl[])
      n2685 = Bundle By Name("t0"=w4350, "Y"=w4359, "dt"=w4354) -> (w4360:waveform(dbl))  [unwired: 1 out]
      n2686 = Set Waveform Attribute(5:w4355, 6:w4356, 7:w4360) -> (3:w4357:waveform(dbl))  [unwired: 1 in, 2 out]
    }
    "APD Display Period (s)" <- w3751
    n2687 = Reciprocal(x=w3751) -> (1/x=→"APD Display Freq. (Hz)":dbl)
    n2688 = local read "Display Period (s)"() -> (w3634:dbl)
    n2689 = Increment(x=w3736) -> (x+1=w3737:dbl)
    n2690 = To Double Precision Float(number=w3646) -> (double precision float=w3645:dbl[])
    n2691 = Index Array(array=w3486, index=0) -> (element=w3490:waveform(dbl))
    n2692 = Index Array(array=w3486, index=1) -> (element=w3485:waveform(dbl))
    n2693 = feedback #11(w3737) -> (w3740:dbl)
    n2694 = Select(t=0, s=w3727, f=w3740) -> (s? t:f=w3733:dbl)
    n2695 = Array Size(array=w3645) -> (size(s)=w3739:i32)
    n2696 = Add(x=w3739, y=w3733) -> (x+y=w3734:dbl)
    n2697 = Unbundle By Name(w3490) -> ("Y"=w3491:dbl[])
    n2698 = feedback #12(w3646) -> (w3723:u32[])
    n2699 = Build Array (concatenate)(w3723, w3646) -> (w3720:u32[])
    n2700 = feedback #13(w3590) -> (w3609:u32[])
    n2701 = Divide(x="Bead Sep. Int. Time (s)", y=w3634) -> (x/y=w3526:dbl)
    n2702 = Build Array (concatenate)(w3609, w3590) -> (w3608:u32[])
    n2703 = Add(x=w3491, y="FB Trap Pos Offset") -> (x+y=w3489:dbl[])
    "T1 x pos data" <- w3489
    n2704 = Greater?(x=w3734, y=w3736) -> (0:w3735:bool)
    n2705 = feedback #14(w3489) -> (w3528:dbl[])
    n2706 = Build Array (concatenate)(w3489, w3528) -> (w3527:dbl[])
    n2707 = Bundle By Name(cluster=w3490, "Y"=w3489) -> (w3488:waveform(dbl))
    n2708 = Select(t=w3733, s=w3735, f=w3734) -> (s? t:f=w3732:dbl)
    n2709 = feedback-in #11(w3732) -> ()
    n2710 = Array Size(array=w3720) -> (size(s)=w3717:i32)
    n2711 = Array Size(array=w3646) -> (size(s)=w3719:i32)
    n2712 = local read "MCL Scanning"() -> (w3730:bool)
    n2713 = local read "APD Integration Time (s)"() -> (w3617:dbl)
    n2714 = Bundle(w3488, w3485) -> (w3484:cluster{waveform(dbl), waveform(dbl)})  [unwired: 1 out]
    n2715 = Build Array (concatenate)(w3610, w3756) -> (w3612:waveform(dbl)[])
    "All Signals" <- w3612
    n2716 = Split 1D Array(array=w3527, index=w3526) -> (first subarray=w3520:dbl[])  [unwired: 1 out]
    n2717 = feedback-in #14(w3520) -> ()
    n2718 = Multiply(x=w3719, y="APD Ave N") -> (x*y=w3718:dbl)
    n2719 = Greater?(x=w3717, y=w3718) -> (0:w3721:bool)
    n2720 = Not(x=w3735) -> (.not. x?=w3729:bool)
    n2721 = Cluster To Array(cluster=w3484) -> (array=w3460:waveform(dbl)[])
    "Trap Positions" <- w3460
    n2722 = To Double Precision Float(number=w3590) -> (double precision float=w3589:dbl[])
    n2723 = call-poly <vilib>:"Mean.vi"("X"=w3520) -> ("mean"=w3519:dbl)  [unwired: 1 out]
    "Mean T1 Position (nm)" <- w3519
    n2724 = Subtract(x=w3520, y=w3519) -> (x-y=w3525:dbl[])
    n2725 = Square(x=w3525) -> (x^2=w3524:dbl[])
    n2726 = And(x=w3729, y=w3730) -> (x .and. y?=w3731:bool)
    n2727 = call-poly <vilib>:"Mean.vi"("X"=w3524) -> ("mean"=w3523:dbl)  [unwired: 1 out]
    n2728 = case shown="True" w3721 {
      tunnel: w3720 -> [w4133 w4140]
      tunnel: [w4133 w4138] -> w3663
      tunnel: w3718 -> [_ w4135]
      tunnel: w3717 -> [_ w4139]
      tunnel: w3608 -> [w4132 w4137]
      tunnel: [w4132 w4134] -> w3605
      frame False {
      }
      frame True {
        n2729 = Subtract(x=w4139, y=w4135) -> (x-y=w4136:dbl)
        n2730 = Array Subset(array=w4140, index=w4136, length=w4135) -> (w4138:u32[])
        n2731 = Array Subset(array=w4137, index=w4136, length=w4135) -> (w4134:u32[])
      }
    }
    n2732 = feedback-in #12(w3663) -> ()
    n2733 = feedback-in #13(w3605) -> ()
    n2734 = Square Root(x=w3523) -> (sqrt(x)=w3522:dbl)
    n2735 = Or(x=w3731, y=w3727) -> (x .or. y?=w3728:bool)
    n2736 = Equal?(x="Tab Control 6", y=T35."High Res Display") -> (x = y?=w3652:bool)
    n2737 = Multiply(x="APD Disp. Scale", y=w3610) -> (x*y=w3619:waveform(dbl)[])
    n2738 = Multiply(x=10.0, y=w3522) -> (x*y=→"Trap 1 Position RMS (A)":dbl)
    n2739 = Multiply(x="APD Disp. Downsample", y=w3617) -> (x*y=w3615:dbl)
    n2740 = Divide(x=w3619, y=w3615) -> (x/y=w3587:waveform(dbl)[])
    n2741 = case "For displaying the high resolution display (no downsampling)" shown="True" w3652 {
      tunnel: w3614 -> [_ w4033]
      frame False {
      }
      frame True {
        n2742 = Index Array(array=w4033, index="High Res. Display") -> (element=w4034:waveform(dbl))
        n2743 = call <vilib>:"Std Deviation and Variance.vi"("X"=w4034) -> ("mean"=w4041:dbl, "standard deviation"=w4046:dbl)  [unwired: 1 in, 1 out]
        "Mean Intensity" <- w4041
        "Sigma" <- w4046
        n2744 = Subtract(x=w4034, y=w4041) -> (x-y=w4040:waveform(dbl))
        n2745 = Select(t=w4040, s="Subtract mean", f=w4034) -> (s? t:f=→"1 Channel":waveform(dbl))
        n2746 = Divide(x=w4046, y=w4041) -> (x/y=→"Sigma/Mean":dbl)
        n2747 = feedback #15(1) -> (w4035:i32)
        n2748 = Greater Or Equal?(x=w4035, y="Slow mean N ave.") -> (x >= y?=w4048:bool)
        n2749 = Increment(x=w4035) -> (x+1=w4050:i32)
        n2750 = Select(t=1, s=w4048, f=w4050) -> (s? t:f=w4037:i32)
        n2751 = feedback-in #15(w4037) -> ()
        n2752 = feedback #16() -> (w4038:waveform(dbl))  [unwired: 1 out]
        n2753 = case shown="Default" w4035 {
          tunnel: [w4053 w4056] -> w4039
          tunnel: w4038 -> [w4055 _]
          tunnel: w4034 -> [w4054 w4056]
          frame Default {
            n2754 = call-poly <vilib>:"Append Waveforms.vi"("waveform B"=w4054, "waveform A"=w4055) -> ("waveform out"=w4053:waveform(dbl))  [unwired: 1 in, 8 out]
          }
          frame 1 {
          }
        }
        n2755 = feedback-in #16(w4039) -> ()
        n2756 = case shown="True" w4048 {
          tunnel: w4039 -> [_ w4052]
          frame False {
          }
          frame True {
            n2757 = call-poly <vilib>:"Mean.vi"("X"=w4052) -> ("mean"=→"Slow mean":dbl)  [unwired: 1 out]
          }
        }
      }
    }
    n2758 = Index Array(array=w3587, index=0) -> (element=w3597:waveform(dbl))
    n2759 = Index Array(array=w3587, index=1) -> (element=w3595:waveform(dbl))
    n2760 = case "For computing FFTs for display" shown="True" "Compute FFT" {
      tunnel: w3614 -> [_ w4747]
      frame False {
      }
      frame True {
        n2761 = Build Array("FFT 1 Choice 1", "FFT 1 Choice 2", "FFT 2 Choice 1", "FFT 2 Choice 2") -> (w4740:u16[])
        n2762 = Array Size(array=w4747) -> (size(s)=w4746:i32)
        n2763 = feedback-in #17(w4740) -> ()
        n2764 = feedback #17(u16[] [100, 100, 100, 100]) -> (w4741:u16[])
        n2765 = feedback-in #18("# Spectra to Ave.") -> ()
        n2766 = feedback #18("# Spectra to Ave.") -> (w4738:dbl)
        n2767 = Not Equal?(x="# Spectra to Ave.", y=w4738) -> (x != y?=w4737:bool)
        n2768 = Not Equal?(x=w4740, y=w4741) -> (x != y?=w4739:bool)
        n2769 = feedback #19(1.0) -> (w4724:dbl)
        n2770 = Compound Arithmetic op=OR("Reset FFT", w4739, w4737) -> (w4722:bool)
        n2771 = Select(t=1.0, s=w4722, f=w4724) -> (s? t:f=w4726:dbl)
        n2772 = Greater?(x=w4726, y="# Spectra to Ave.") -> (0:w4745:bool)
        n2773 = Increment(x=w4726) -> (x+1=w4725:dbl)
        n2774 = feedback-in #19(w4725) -> ()
        n2775 = local read "DMA Update Period (s)"() -> (w4720:dbl)
        n2776 = Multiply(x="# Spectra to Ave.", y=w4720) -> (x*y=→"Ave. Time (s)":dbl)
        n2777 = Build Array(cluster{"f0":dbl, "df":dbl, "magnitude":dbl[]} {"f0"=0.0, "df"=0.0, "magnitude"=[]} ("PSD")) -> (w4729:cluster{"f0":dbl, "df":dbl, "magnitude":dbl[]}[])
        n2778 = Build Array(w4729, w4729, w4729, w4729) -> (w4731:T46)
        n2779 = feedback #20(w4731) -> (w4736:T46)
        n2780 = for {
          N: 4 -> [_]
          tunnel: w4740 -> [w4769] mode=indexing
          tunnel: w4747 -> [w4770]
          tunnel: w4746 -> [w4772]
          tunnel: w4722 -> [w4765]
          tunnel: w4745 -> [w4764]
          tunnel: "# Spectra to Ave." -> [w4763]
          tunnel: [w4762] -> w4735 mode=indexing
          tunnel: w4736 -> [w4767] mode=indexing
          tunnel: [w4766] -> w4723 mode=indexing
          tunnel: w4726 -> [w4761]
          n2781 = Less?(x=w4769, y=w4772) -> (x < y?=w4771:bool)
          n2782 = Index Array(array=w4770, index=w4769) -> (element=w4768:waveform(dbl))
          n2783 = case shown="True" w4771 {
            tunnel: w4768 -> [_ w4789]
            tunnel: w4767 -> [w4774 w4787]
            tunnel: [w4774 w4775] -> w4766
            tunnel: w4765 -> [_ w4786]
            tunnel: w4764 -> [_ w4779]
            tunnel: w4763 -> [_ w4778]
            tunnel: [cluster{"f0":dbl, "df":dbl, "magnitude":dbl[]} {"f0"=0.0, "df"=0.0, "magnitude"=[]} ("PSD") w4780] -> w4762
            tunnel: w4761 -> [_ w4777]
            frame False {
            }
            frame True {
              n2784 = call <vilib>:"Std Deviation and Variance.vi"("X"=w4789) -> ("mean"=w4790:dbl)  [unwired: 1 in, 2 out]
              n2785 = Subtract(x=w4789, y=w4790) -> (x-y=w4788:waveform(dbl))
              n2786 = xnode "Spectral Measurements"("Signals"=w4788) -> ("PSD"=w4782:cluster{"f0":dbl, "df":dbl, "magnitude":dbl[]})  [unwired: 1 in, 1 out]
              n2787 = case shown="False" w4786 {
                tunnel: w4787 -> [w4799 _]
                tunnel: [w4795 w4804] -> w4775
                tunnel: w4782 -> [w4798 w4805]
                tunnel: w4779 -> [w4797 _]
                frame False {
                  n2788 = Build Array (concatenate)(w4799, w4798) -> (w4796:cluster{"f0":dbl, "df":dbl, "magnitude":dbl[]}[])
                  n2789 = case shown="True" w4797 {
                    tunnel: w4796 -> [w4800 w4803]
                    tunnel: [w4800 w4801] -> w4795
                    frame False {
                    }
                    frame True {
                      n2790 = Delete From Array(array=w4803, index=0) -> (array with subset deleted=w4801:cluster{"f0":dbl, "df":dbl, "magnitude":dbl[]}[])  [unwired: 1 in, 1 out]
                    }
                  }
                }
                frame True {
                  n2791 = Build Array(w4805) -> (w4804:cluster{"f0":dbl, "df":dbl, "magnitude":dbl[]}[])
                }
              }
              n2792 = for {
                tunnel: w4775 -> [w4794] mode=indexing
                tunnel: [w4793] -> w4785 mode=indexing
                workers-P: _ -> [_]
                n2793 = Unbundle By Name(w4794) -> ("magnitude"=w4793:dbl[])
              }
              n2794 = Transpose 2D Array(2D array=w4785) -> (transposed array=w4784:dbl[][])
              n2795 = for {
                tunnel: w4784 -> [w4792] mode=indexing
                tunnel: [w4791] -> w4783 mode=indexing
                workers-P: _ -> [_]
                n2796 = Add Array Elements(numeric array=w4792) -> (sum=w4791:dbl)
              }
              n2797 = Select(t=w4778, s=w4779, f=w4777) -> (s? t:f=w4776:dbl)
              n2798 = Divide(x=w4783, y=w4776) -> (x/y=w4781:dbl[])
              n2799 = Bundle By Name(cluster=w4782, "magnitude"=w4781) -> (w4780:cluster{"f0":dbl, "df":dbl, "magnitude":dbl[]})
            }
          }
        }
        n2800 = case shown="True" w4722 {
          tunnel: w4723 -> [w4754 w4760]
          tunnel: [w4754 w4755] -> w4721
          frame False {
          }
          frame True {
            n2801 = Array Subset(array=w4760, index (row)=0 ("index"), length (row)=4 ("length"), index (col)=0 ("index"), length (col)=1 ("length")) -> (w4755:T46)
          }
        }
        n2802 = feedback-in #20(w4721) -> ()
        n2803 = Split 1D Array(array=w4735, index=2) -> (first subarray=→"FFT 1":cluster{"f0":dbl, "df":dbl, "magnitude":dbl[]}[], second subarray=→"FFT 2":cluster{"f0":dbl, "df":dbl, "magnitude":dbl[]}[])
      }
    }
    n2804 = case "For plotting results of scanning MCL" shown="True" w3728 {
      tunnel: w3727 -> [_ w4173]
      tunnel: w3645 -> [_ w4269]
      tunnel: w3736 -> [_ _]
      tunnel: w3614 -> [_ w4243]
      tunnel: w3589 -> [_ w4174]
      tunnel: w3588 -> [_ w4147]
      frame False {
      }
      frame True {
        w4154 = u32 0 items=["Horizontal", "Vertical", "Central", "1st Diagonal", "2nd Diagonal"] ("Type of Symmetry")
        w4182 = u32 0 items=["Horizontal", "Vertical", "Central", "1st Diagonal", "2nd Diagonal"] ("Type of Symmetry")
        w4185 = u32 0 items=["Horizontal", "Vertical", "Central", "1st Diagonal", "2nd Diagonal"] ("Type of Symmetry")
        w4214 = u32 0 items=["Horizontal", "Vertical", "Central", "1st Diagonal", "2nd Diagonal"] ("Type of Symmetry")
        n2805 = Index Array(array=w4243, index=10) -> (element=w4249:waveform(dbl))
        n2806 = Index Array(array=w4243, index=11) -> (element=w4246:waveform(dbl))
        n2807 = local read "Cycles/step (MCL)"() -> (w4199:u64)
        n2808 = Index Array(array=w4243, index="Channel") -> (element=w4245:waveform(dbl))
        n2809 = Unbundle(w4147) -> ("New Image"=w4146:T2, "New Image"=w4145:T2, "New Image"=w4144:T2, "New Image"=w4143:T2)
        n2810 = Unbundle By Name(w4249) -> ("Y"=w4201:dbl[])
        n2811 = Unbundle By Name(w4246) -> ("Y"=w4203:dbl[])
        n2812 = Unbundle By Name(w4245) -> ("Y"=w4208:dbl[])
        n2813 = call "downsample 1D array - double.vi"("Ave N"=w4199, "Array In"=w4201) -> ("Array Out"=w4200:dbl[])  [unwired: 1 out]
        n2814 = call "downsample 1D array - double.vi"("Ave N"=w4199, "Array In"=w4203) -> ("Array Out"=w4202:dbl[])  [unwired: 1 out]
        n2815 = call "downsample 1D array - double.vi"("Ave N"=w4199, "Array In"=w4208) -> ("Array Out"=w4207:dbl[])  [unwired: 1 out]
        n2816 = feedback #21(w4269) -> (w4270:dbl[])
        n2817 = Build Array (concatenate)(w4270, w4269) -> (w4251:dbl[])
        n2818 = feedback #22(w4174) -> (w4176:dbl[])
        n2819 = Build Array (concatenate)(w4176, w4174) -> (w4175:dbl[])
        n2820 = local read "Scan steps (MCL)"() -> (w4156:u64)
        n2821 = Select(t=w4269, s=w4173, f=w4251) -> (s? t:f=w4255:dbl[])
        n2822 = feedback-in #21(w4255) -> ()
        n2823 = Select(t=w4174, s=w4173, f=w4175) -> (s? t:f=w4157:dbl[])
        n2824 = feedback-in #22(w4157) -> ()
        n2825 = local read "Scan lines (y)"() -> (w4142:u64)
        n2826 = local read "N APD Samp/step"() -> (w4158:dbl)
        n2827 = feedback #23(w4200) -> (w4257:dbl[])
        n2828 = Build Array (concatenate)(w4257, w4200) -> (w4248:dbl[])
        n2829 = feedback #24(w4207) -> (w4267:dbl[])
        n2830 = Build Array (concatenate)(w4267, w4207) -> (w4266:dbl[])
        n2831 = feedback #25(w4202) -> (w4259:dbl[])
        n2832 = Build Array (concatenate)(w4259, w4202) -> (w4260:dbl[])
        n2833 = Select(t=w4200, s=w4173, f=w4248) -> (s? t:f=w4204:dbl[])
        n2834 = feedback-in #23(w4204) -> ()
        n2835 = Select(t=w4207, s=w4173, f=w4266) -> (s? t:f=w4206:dbl[])
        n2836 = feedback-in #24(w4206) -> ()
        n2837 = Select(t=w4202, s=w4173, f=w4260) -> (s? t:f=w4205:dbl[])
        n2838 = feedback-in #25(w4205) -> ()
        n2839 = Multiply(x=w4156, y=u64 2) -> (x*y=w4141:u64)
        n2840 = call "integrate 1D array interval - double.vi"("Ave N"=w4158, "Array In"=w4157) -> ("Array Out"=w4169:dbl[])  [unwired: 1 out]
        n2841 = call "integrate 1D array interval - double.vi"("Ave N"=w4158, "Array In"=w4255) -> ("Array Out"=w4254:dbl[])  [unwired: 1 out]
        n2842 = Array Size(array=w4169) -> (size(s)=w4170:i32)
        n2843 = Array Size(array=w4254) -> (size(s)=w4256:i32)
        n2844 = Multiply(x=w4142, y=w4141) -> (x*y=w4172:u64)
        n2845 = Multiply(x=w4142, y=w4141) -> (x*y=w4264:u64)
        n2846 = call-poly <vilib>:"Mean.vi"("X"=w4204) -> ("mean"=w4188:dbl)  [unwired: 1 out]
        n2847 = Subtract(x=w4172, y=w4170) -> (x-y=w4163:u64)
        n2848 = call-poly <vilib>:"Mean.vi"("X"=w4206) -> ("mean"=w4193:dbl)  [unwired: 1 out]
        n2849 = call-poly <vilib>:"Mean.vi"("X"=w4205) -> ("mean"=w4191:dbl)  [unwired: 1 out]
        n2850 = call-poly <vilib>:"Mean.vi"("X"=w4169) -> ("mean"=w4160:dbl)  [unwired: 1 out]
        n2851 = Subtract(x=w4264, y=w4256) -> (x-y=w4198:u64)
        n2852 = call-poly <vilib>:"Mean.vi"("X"=w4254) -> ("mean"=w4195:dbl)  [unwired: 1 out]
        n2853 = Initialize Array(1.0 ("element"), w4163) -> (w4159:dbl[])
        n2854 = Initialize Array(1.0 ("element"), w4198) -> (w4189:dbl[])
        n2855 = Multiply(x=w4159, y=w4160) -> (x*y=w4161:dbl[])
        n2856 = Multiply(x=w4189, y=w4191) -> (x*y=w4192:dbl[])
        n2857 = Multiply(x=w4189, y=w4193) -> (x*y=w4194:dbl[])
        n2858 = Multiply(x=w4189, y=w4188) -> (x*y=w4190:dbl[])
        n2859 = Multiply(x=w4189, y=w4195) -> (x*y=w4196:dbl[])
        n2860 = Build Array (concatenate)(w4204, w4190) -> (w4258:dbl[])
        n2861 = Build Array (concatenate)(w4206, w4194) -> (w4262:dbl[])
        n2862 = Build Array (concatenate)(w4205, w4192) -> (w4261:dbl[])
        n2863 = Build Array (concatenate)(w4169, w4161) -> (w4171:dbl[])
        n2864 = Build Array (concatenate)(w4254, w4196) -> (w4263:dbl[])
        n2865 = Reshape Array(w4258, w4142, w4141) -> (w4224:dbl[][])
        n2866 = Reshape Array(w4171, w4142, w4141) -> (w4167:dbl[][])
        n2867 = Reshape Array(w4262, w4142, w4141) -> (w4216:dbl[][])
        n2868 = Reshape Array(w4261, w4142, w4141) -> (w4231:dbl[][])
        n2869 = Reshape Array(w4263, w4142, w4141) -> (w4241:dbl[][])
        n2870 = Array Subset(array=w4231, index (col)=0 ("index"), length (col)=w4156) -> (w4236:dbl[][])  [unwired: 2 in]
        n2871 = Array Subset(array=w4231, index (col)=w4156) -> (w4234:dbl[][])  [unwired: 3 in]
        n2872 = Array Subset(array=w4216, index (col)=0 ("index"), length (col)=w4156) -> (w4222:dbl[][])  [unwired: 2 in]
        n2873 = Array Subset(array=w4216, index (col)=w4156) -> (w4220:dbl[][])  [unwired: 3 in]
